vi "Read Busy Flag and Address.vi"(6 "chip select  (1st chip)":enum16{"1st chip", "2nd chip"}(ring), 8 "error in (no error)":errorcluster, 11 "HD44780 in":refnum<class "HD44780.lvclass">) -> (0 "error out":errorcluster, 1 "address":u8=97 format="%.0x", 2 "busy flag":bool, 3 "HD44780 out":refnum<class "HD44780.lvclass">)   [LabVIEW 2017, in "HD44780.lvclass"]
uses:
  HD44780.lvclass
  HD44780.lvclass/HD44780.ctl
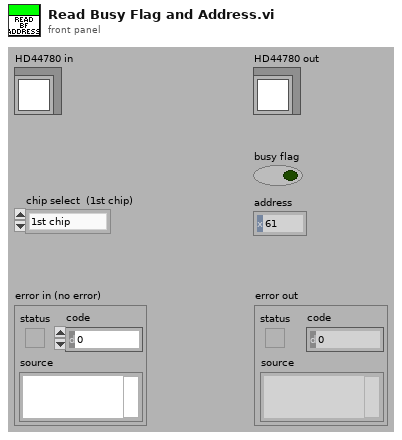
[diagram p1: front panel]
types:
  T1 = typedef "HD44780 Common.lvlib/cluster of class private data.ctl" = cluster{"FPGA VI Reference":refnum<k20>, "device index":i8, "screen size":T2, "font size":T3, "auto wrap":bool, "alignment":T4, "number of line":T5, "shift 0":i8, "entry mode 0":T6, "shift 1":i8, "entry mode 1":T6}
  T2 = typedef "HD44780 Common.lvlib/screen size.ctl" = enum8{"8x1", "8x2", "12x4", "16x1", "16x2", "16x4", "20x1", "20x2", "20x4", "24x1", "24x2", "40x2", "40x4"}
  T3 = typedef "HD44780 Common.lvlib/font size.ctl" = enum8{"5x8", "5x10"}
  T4 = typedef "HD44780 Common.lvlib/alignment.ctl" = enum16{"None", "Left", "Center", "Right"}
  T5 = typedef "HD44780 Common.lvlib/line number.ctl" = enum8{"1 line", "2 lines"}
  T6 = typedef "HD44780 Common.lvlib/entry mode.ctl" = enum8{"increment & no shift", "increment & shift", "decrement & no shift", "decrement & shift"}
  T7 = cluster{"FPGA VI Reference":refnum<k20>, "device index":i8, "screen size":enum8{"8x1", "8x2", "12x4", "16x1", "16x2", "16x4", "20x1", "20x2", "20x4", "24x1", "24x2", "40x2", "40x4"}, "font size":enum8{"5x8", "5x10"}, "auto wrap":bool, "alignment":enum16{"None", "Left", "Center", "Right"}, "number of line":enum8{"1 line", "2 lines"}, "shift 0":i8, "entry mode 0":enum8{"increment & no shift", "increment & shift", "decrement & no shift", "decrement & shift"}, "shift 1":i8, "entry mode 1":enum8{"increment & no shift", "increment & shift", "decrement & no shift", "decrement & shift"}}
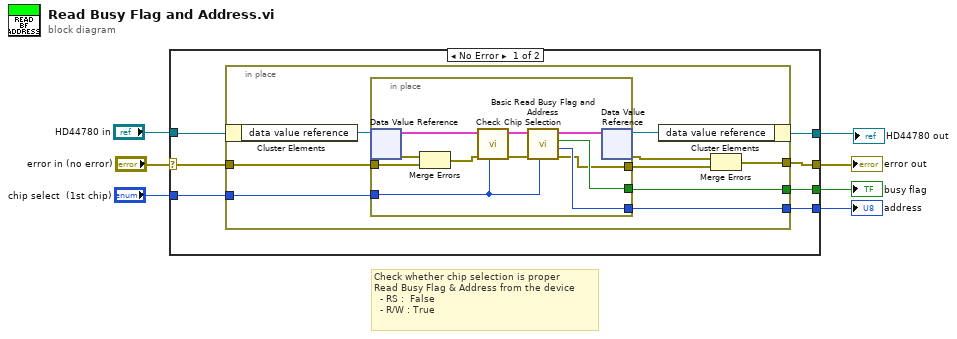
[diagram p0: block diagram]
diagram:
  # "Check whether chip selection is proper\nRead Busy Flag & Address from the device\n  - RS :  False \n  - R/W : True"
  n1 = case shown="No Error" "error in (no error)" {
    selector: "error in (no error)" -> [w11 w36]
    tunnel: "chip select  (1st chip)" -> [w14 _]
    tunnel: "HD44780 in" -> [w10 w35]
    tunnel: [w13 _] -> w5
    tunnel: [w12 _] -> w4
    tunnel: [w9 w36] -> w3
    tunnel: [w8 w35] -> w1
    frame No Error {
      n2 = in-place {
        in-place-border: w14 -> [w23]
        in-place-border: [w22] -> w13
        in-place-border: [w21] -> w12
        in-place-border: w11 -> [w20]
        in-place-border: [w15] -> w9
        n3 = in-place-cluster #1(w10) -> ("data value reference"=w19:refnum<data-value>)
        n4 = in-place {
          in-place-border: w23 -> [w24]
          in-place-border: [w34] -> w22
          in-place-border: [w33] -> w21
          in-place-border: [w32] -> w16
          in-place-border: w20 -> [w30]
          n5 = in-place-dvr #2(w19) -> (w28:T1, w31:errorcluster)
          n6 = Merge Errors(w31, w30) -> (w26:errorcluster)
          n7 = call "Check Chip Selection.vi"("chip select"=w24, "error in (no error)"=w26, "cluster of private data in"=w28) -> ("error out"=w25:errorcluster, "cluster of private data out"=w27:T7)  [unwired: 7 in]
          n8 = call "Basic Read Busy Flag and Address.vi"("chip select  (1st chip)"=w24, "error in (no error)"=w25, "cluster of private data in"=w27) -> ("error out"=w32:errorcluster, "address"=w33:u8, "busy flag"=w34:bool, "cluster of private data out"=w29:T7)  [unwired: 5 in]
          n9 = in-place-dvr #2(w29) -> (w18:refnum<data-value>, w17:errorcluster)
        }
        n10 = in-place-cluster #1("data value reference"=w18) -> (w8:refnum<class "HD44780.lvclass">)
        n11 = Merge Errors(w17, w16) -> (w15:errorcluster)
      }
    }
    frame Error {
    }
  }
  "error out" <- w3
  "HD44780 out" <- w1
  "busy flag" <- w5
  "address" <- w4
